vi "Sondenmodell.InitObject.vi"(8 "Error In":errorcluster, 11 "ModelMainPath":path) -> (0 "Error out":errorcluster, 3 "Sondenmodell":refnum<data-value>)   [LabVIEW 2016, in "Sondenmodell.lvclass"]
uses:
  Sondenmodell.lvclass
  Package ResourceControl/ObjectHandler/ObjectHandler.GetObjectWType.ctl
  Package ResourceControl/ObjectHandler/ObjectHandler.ObjectType.ctl
  Package ResourceControl/ObjectHandler/ObjectHandler.ObjectMessage.ctl
  Package ResourceControl/ObjectHandler/ObjectHandler.ObjectWType.ctl
  Package ResourceControl/ObjectHandler/ObjectHandler.lvclass
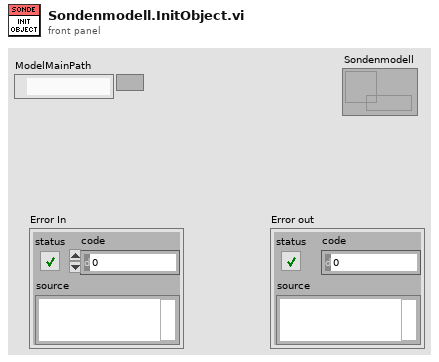
[diagram p1: front panel]
types:
  T1 = typedef "ObjectHandler.lvclass/ObjectHandler.ObjectMessage.ctl" = cluster{"Name":string, "ObjectWType":T2}
  T2 = typedef "ObjectHandler.lvclass/ObjectHandler.ObjectWType.ctl" = cluster{"ObjectType":T3, "Object":variant}
  T3 = typedef "ObjectHandler.lvclass/ObjectHandler.ObjectType.ctl" = enum16{"undefined", "ObjectHandler", "ViHandler", "ErrorHandler", "CentralStorage", "Hausmodell", "Sondenmodell", "Wärmepumpe", "Umgebung"}
  T4 = typedef "ObjectHandler.lvclass/ObjectHandler.GetObjectWType.ctl" = cluster{"Name":string, "Caller":string}
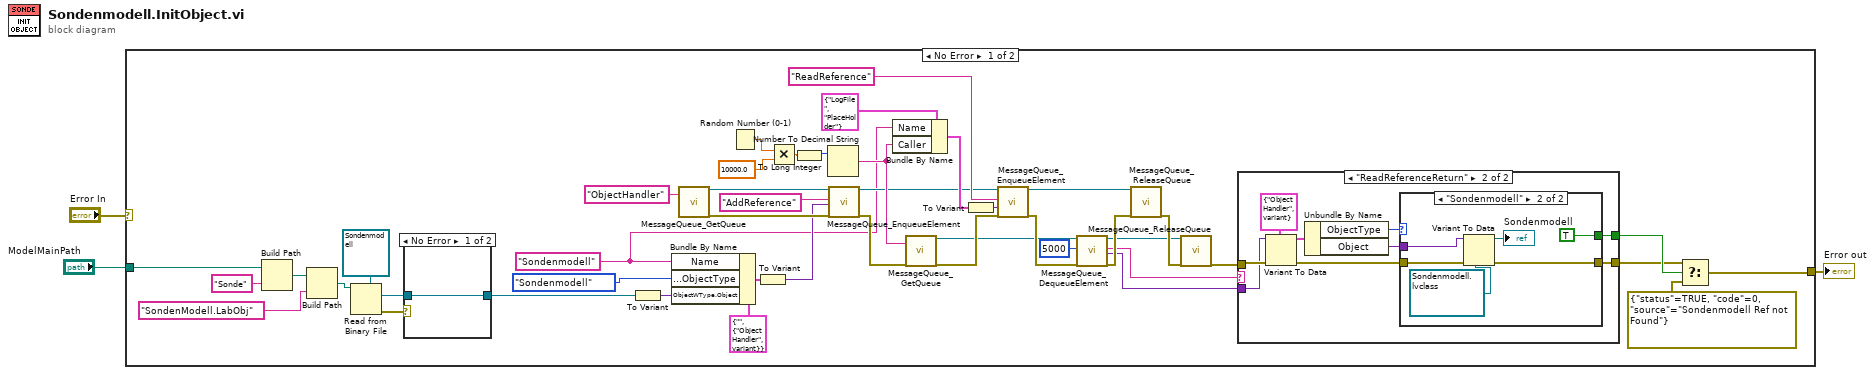
[diagram p0: block diagram]
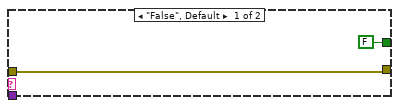
[diagram p2: hidden frame]
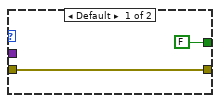
[diagram p3: hidden frame]
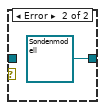
[diagram p4: hidden frame]
diagram:
  n1 = case shown="No Error" "Error In" {
    selector: "Error In" -> [_ w70]
    tunnel: [w48 w70] -> w3
    tunnel: "ModelMainPath" -> [w7 _]
    frame No Error {
      w13 = "Sondenmodell" ("Name")
      n2 = Build Path(base path=w7, name or relative path="Sonde") -> (appended path=w10:path)
      n3 = Build Path(base path=w10, name or relative path="SondenModell.LabObj") -> (appended path=w12:path)
      n4 = Read from Binary File(5:refnum<class "Sondenmodell.lvclass"> refnum ("Sondenmodell.lvclass"), 11:w12) -> (0:w6:errorcluster, 2:w4:refnum<class "Sondenmodell.lvclass">)  [unwired: 4 in, 2 out]
      n5 = case shown="No Error" w6 {
        tunnel: [w68 refnum<class "Sondenmodell.lvclass"> refnum ("Sondenmodell.lvclass")] -> w5
        tunnel: w4 -> [w68 _]
        frame No Error {
        }
        frame Error {
        }
      }
      n6 = To Variant(anything=w5) -> (Variant=w20:variant)
      n7 = Bundle By Name(cluster=T1 {"Name"="", "ObjectWType"={"ObjectType"=enum."ObjectHandler", "Object"=variant(refnum<data-value> refnum)}} ("ObjectMessage"), "Name"=w13, "ObjectWType.ObjectType"=ObjectHandler.ObjectType."Sondenmodell" ("ObjectType"), "ObjectWType.Object"=w20) -> (w19:T1)
      n8 = call "MessageQueue_GetQueue.vi"("Name"="ObjectHandler") -> ("QueueOut"=w22:refnum<queue>, "ErrorOut"=w23:errorcluster)  [unwired: 16 in, 1 out]
      n9 = Random Number (0-1)() -> (number: 0 to 1=w47:dbl)
      n10 = To Variant(anything=w19) -> (Variant=w18:variant)
      n11 = Multiply(x=w47, y=10000.0) -> (x*y=w45:dbl)
      n12 = To Long Integer(number=w45) -> (32bit integer=w44:i32)
      n13 = Number To Decimal String(number=w44) -> (decimal integer string=w29:string)  [unwired: 1 in]
      n14 = call "MessageQueue_EnqueueElement.vi"("QueueIn"=w22, "Message"="AddReference", "Data"=w18, "ErrorIn"=w23) -> ("QueueOut"=w14:refnum<queue>, "ErrorOut"=w15:errorcluster)  [unwired: 14 in]
      n15 = Bundle By Name(cluster=T4 {"Name"="LogFile", "Caller"="PlaceHolder"} ("GetRefInput"), "Name"=w13, "Caller"=w29) -> (w28:T4)
      n16 = call "MessageQueue_GetQueue.vi"("Name"=w29, "ErrorIn"=w15) -> ("QueueOut"=w38:refnum<queue>, "ErrorOut"=w43:errorcluster)  [unwired: 15 in, 1 out]
      n17 = To Variant(anything=w28) -> (Variant=w33:variant)
      n18 = call "MessageQueue_EnqueueElement.vi"("QueueIn"=w14, "Message"="ReadReference", "Data"=w33, "ErrorIn"=w43) -> ("QueueOut"=w39:refnum<queue>, "ErrorOut"=w42:errorcluster)  [unwired: 14 in]
      n19 = call "MessageQueue_DequeueElement.vi"("QueueIn"=w38, "Timeout"=5000, "ErrorIn"=w42) -> ("QueueOut"=w37:refnum<queue>, "Message"=w35:string, "Data"=w31:variant, "ErrorOut"=w41:errorcluster)  [unwired: 12 in, 1 out]
      n20 = call "MessageQueue_ReleaseQueue.vi"("QueueIn"=w39, "ErrorIn"=w41) -> ("ErrorOut"=w40:errorcluster)  [unwired: 15 in, 2 out]
      n21 = call "MessageQueue_ReleaseQueue.vi"("QueueIn"=w37, "ErrorIn"=w40) -> ("ErrorOut"=w32:errorcluster)  [unwired: 15 in, 2 out]
      n22 = case shown="\"ReadReferenceReturn\"" w35 {
        tunnel: w32 -> [w49 w59]
        tunnel: w31 -> [_ w58]
        tunnel: [w49 w52] -> w26
        tunnel: [FALSE w51] -> w27
        frame "False", Default {
        }
        frame "ReadReferenceReturn" {
          n23 = Variant To Data(error in=w59, type=T2 {"ObjectType"=enum."ObjectHandler", "Object"=variant} ("ObjectWType"), Variant=w58) -> (data=w56:T2, error out=w53:errorcluster)
          n24 = Unbundle By Name(w56) -> ("ObjectType"=w55:T3, "Object"=w54:variant)
          n25 = case shown="\"Sondenmodell\"" w55 {
            tunnel: w54 -> [_ w67]
            tunnel: w53 -> [w61 w66]
            tunnel: [w61 w65] -> w52
            tunnel: [FALSE TRUE] -> w51
            frame Default {
            }
            frame "Sondenmodell" {
              n26 = Variant To Data(error in=w66, type=refnum<data-value> refnum ("data value reference"), Variant=w67) -> (data=→"Sondenmodell":refnum<data-value>, error out=w65:errorcluster)
            }
          }
        }
      }
      n27 = Select(t=w26, s=w27, f=errorcluster {"status"=TRUE, "code"=0, "source"="Sondenmodell Ref not Found"}) -> (s? t:f=w48:errorcluster)
    }
    frame Error {
    }
  }
  "Error out" <- w3
